vi "meas_1_lxy.vi"(0 "config":T1={"initialize"=enum."SR830", "6221"={"6221 Resource"="GPIB0::24::INSTR", "Delta status"=FALSE, "电流|RMS(A)"=0.0}, "SR830+6221"={"source"=0, "Current(A)"=0.0, "阻抗(Ohm)"=0.0, "SR830 1"=FALSE, "SR830 2"=FALSE, "SR830 3"=FALSE, "SR830 4"=FALSE, "VISA 1"="", "VISA 2"="", "VISA 3"="", "VISA 4"="", "Reserve 1"=0, "Reserve 2"=-1, "Reserve 3"=-1, "Reserve 4"=-1, "Sensitivity 1"=-1, "Sensitivity 2"=0, "Sensitivity 3"=-1, "Sensitivity 4"=-1, "量程入 1"=0, "量程入 2"=0, "量程入 3"=0, "量程入 4"=0}, "2400"={"2400"=FALSE, "VISA"="", "Output Level (0)"=1e-05, "Compliance  Level (0.1)"=10.0, "ch"=[]}, "ch"={"ch"=[], "current"=[], "change?"=[], "holding current\nwhen change ch?"=FALSE, "current offset"=[]}, "Instrument"={"limit"={"Field limit"=0.0, "Field rate limit"=0.0, "Temp limit"=0.0, "Temp low limit"=0.0, "Temp rate limit "=0.0}, "genarl"={"行数"=refnum, "编辑列表框？"=refnum, "列表框"=refnum, "camg 振荡状态"=refnum, "Aborting"=refnum, "数据文件"=refnum, "warning"=refnum, "vi路径"="", "Instrument Type"=enum."PPMS-Rotate"}, "cmag"={"TM620"="TCPIP0::192.168.1.5::4266::SOCKET", "M24C Resource"="GPIB0::24::INSTR", "4G supply"="", "Temp Status 24C"=refnum, "Temp"=refnum, "9T信号"=refnum, "4g supply status"=refnum, "in-plane"="", "out-plane"="", "in-plane signal"=FALSE, "out-plane signal"=FALSE, "in plane 信号"=refnum, "pzt volt"=refnum, "camg Rate"=refnum}, "lengtou2"={"750 visa"="", "750 rotate"="", "semaphore 340"=refnum, "semaphore 750"=refnum, "750 field status"=refnum, "Input (0:A) 340"=0, "340 Resource"="GPIB0::14::INSTR", "340 Status"=refnum, "Input (0:B) 340"=1, "Loop (0: 1)"=0, "Loop (1: 1)"=0, "TCP master instance"=refnum}, "lengtou"={"TCP master instance"=refnum, "335 Status"=refnum, "335 Resource "="GPIB0::24::INSTR", "Input (0:A) 335"=0, "Input (0:B) 335"=1, "Heater Output (1:1) 335"=1, "semaphore 335"=refnum}, "325 for test"={"quantum design"=refnum, "semaphore 325"=refnum, "325 Resource "="GPIB0::13::INSTR", "Input (0:A) 325"=0, "Heater Output (1:1) 325"=1, "325 Status"=refnum}}, "2614B"={"2614B chA"=FALSE, "2614B chB"=FALSE, "VISA"=""}, "33522b"={"33522b resource name"="", "零电压"=0.0, "最大电压"=148.0, "间隔"=4.0, "最小电压"=-48.0, "loop"=0.0, "压电陶瓷电压(Vpp)"=0.0}, "gating type"=enum."2614(daul)", "层数"=0, "行数"=0, "是否处理"=[], "current 2"=[]} {"Instrument"."325 for test"."Heater Output (1:1) 325" items=["1"=1, "2"=2]; "Instrument"."325 for test"."Input (0:A) 325" items=["A", "B"]; "Instrument"."lengtou"."Heater Output (1:1) 335" items=["1"=1, "2"=2]; "Instrument"."lengtou"."Input (0:B) 335" items=["A", "B"]; "Instrument"."lengtou"."Input (0:A) 335" items=["A", "B"]; "Instrument"."lengtou2"."Loop (1: 1)" items=["1", "2"]; "Instrument"."lengtou2"."Loop (0: 1)" items=["1", "2"]; "Instrument"."lengtou2"."Input (0:B) 340" items=["A", "B", "C", "D"]; "Instrument"."lengtou2"."Input (0:A) 340" items=["A", "B", "C", "D"]; "SR830+6221"."Sensitivity 4" items=["Auto Gain"=-1, "2 nV/fA"=0, "5 nV/fA"=1, "10 nV/fA"=2, "20 nV/fA"=3, "50 nV/fA"=4, "100 nV/fA"=5, "200 nV/fA"=6, "500 nV/fA"=7, "1 uV/pA"=8, "2 uV/pA"=9, "5 uV/pA"=10, "10 uV/pA"=11, "20 uV/pA"=12, "50 uV/pA"=13, "100 uV/pA"=14, "200 uV/pA"=15, "500 uV/pA"=16, "1 mV/nA"=17, "2 mV/nA"=18, "5 mV/nA"=19, "10 mV/nA"=20, "20 mV/nA"=21, "50 mV/nA"=22, "100 mV/nA"=23, "200 mV/nA"=24, "500 mV/mA"=25, "1 V/uA"=26]; "SR830+6221"."Sensitivity 3" items=["Auto Gain"=-1, "2 nV/fA"=0, "5 nV/fA"=1, "10 nV/fA"=2, "20 nV/fA"=3, "50 nV/fA"=4, "100 nV/fA"=5, "200 nV/fA"=6, "500 nV/fA"=7, "1 uV/pA"=8, "2 uV/pA"=9, "5 uV/pA"=10, "10 uV/pA"=11, "20 uV/pA"=12, "50 uV/pA"=13, "100 uV/pA"=14, "200 uV/pA"=15, "500 uV/pA"=16, "1 mV/nA"=17, "2 mV/nA"=18, "5 mV/nA"=19, "10 mV/nA"=20, "20 mV/nA"=21, "50 mV/nA"=22, "100 mV/nA"=23, "200 mV/nA"=24, "500 mV/mA"=25, "1 V/uA"=26]; "SR830+6221"."Sensitivity 1" items=["Auto Gain"=-1, "2 nV/fA"=0, "5 nV/fA"=1, "10 nV/fA"=2, "20 nV/fA"=3, "50 nV/fA"=4, "100 nV/fA"=5, "200 nV/fA"=6, "500 nV/fA"=7, "1 uV/pA"=8, "2 uV/pA"=9, "5 uV/pA"=10, "10 uV/pA"=11, "20 uV/pA"=12, "50 uV/pA"=13, "100 uV/pA"=14, "200 uV/pA"=15, "500 uV/pA"=16, "1 mV/nA"=17, "2 mV/nA"=18, "5 mV/nA"=19, "10 mV/nA"=20, "20 mV/nA"=21, "50 mV/nA"=22, "100 mV/nA"=23, "200 mV/nA"=24, "500 mV/mA"=25, "1 V/uA"=26]; "SR830+6221"."Sensitivity 2" items=["Auto Gain"=-1, "2 nV/fA"=0, "5 nV/fA"=1, "10 nV/fA"=2, "20 nV/fA"=3, "50 nV/fA"=4, "100 nV/fA"=5, "200 nV/fA"=6, "500 nV/fA"=7, "1 uV/pA"=8, "2 uV/pA"=9, "5 uV/pA"=10, "10 uV/pA"=11, "20 uV/pA"=12, "50 uV/pA"=13, "100 uV/pA"=14, "200 uV/pA"=15, "500 uV/pA"=16, "1 mV/nA"=17, "2 mV/nA"=18, "5 mV/nA"=19, "10 mV/nA"=20, "20 mV/nA"=21, "50 mV/nA"=22, "100 mV/nA"=23, "200 mV/nA"=24, "500 mV/mA"=25, "1 V/uA"=26]; "SR830+6221"."Reserve 4" items=["Auto Gain"=-1, "2 nV/fA"=0, "5 nV/fA"=1, "10 nV/fA"=2, "20 nV/fA"=3, "50 nV/fA"=4, "100 nV/fA"=5, "200 nV/fA"=6, "500 nV/fA"=7, "1 uV/pA"=8, "2 uV/pA"=9, "5 uV/pA"=10, "10 uV/pA"=11, "20 uV/pA"=12, "50 uV/pA"=13, "100 uV/pA"=14, "200 uV/pA"=15, "500 uV/pA"=16, "1 mV/nA"=17, "2 mV/nA"=18, "5 mV/nA"=19, "10 mV/nA"=20, "20 mV/nA"=21, "50 mV/nA"=22, "100 mV/nA"=23, "200 mV/nA"=24, "500 mV/mA"=25, "1 V/uA"=26]; "SR830+6221"."Reserve 3" items=["Auto Reserve"=-1, "High Reserve"=0, "Normal"=1, "Low Noise"=2]; "SR830+6221"."Reserve 2" items=["Auto Reserve"=-1, "High Reserve"=0, "Normal"=1, "Low Noise"=2]; "SR830+6221"."Reserve 1" items=["Auto Reserve"=-1, "High Reserve"=0, "Normal"=1, "Low Noise"=2]; "SR830+6221"."source" items=["SR830 1", "SR830 2", "SR830 3", "SR830 4"]}, 1 "压电陶瓷电压 (Vpp)":dbl=0.1, 5 "6221ch":i32, 7 "2400通道":i32, 9 "电流（A）":dbl, 11 "错误输入（无错误）":errorcluster, 12 "change？":bool) -> (4 "数组":string[](array[string]), 6 "输出簇":T1={"initialize"=enum."SR830", "6221"={"6221 Resource"="GPIB0::24::INSTR", "Delta status"=FALSE, "电流|RMS(A)"=0.0}, "SR830+6221"={"source"=0, "Current(A)"=0.0, "阻抗(Ohm)"=0.0, "SR830 1"=FALSE, "SR830 2"=FALSE, "SR830 3"=FALSE, "SR830 4"=FALSE, "VISA 1"="", "VISA 2"="", "VISA 3"="", "VISA 4"="", "Reserve 1"=0, "Reserve 2"=-1, "Reserve 3"=-1, "Reserve 4"=-1, "Sensitivity 1"=-1, "Sensitivity 2"=0, "Sensitivity 3"=-1, "Sensitivity 4"=-1, "量程入 1"=0, "量程入 2"=0, "量程入 3"=0, "量程入 4"=0}, "2400"={"2400"=FALSE, "VISA"="", "Output Level (0)"=1e-05, "Compliance  Level (0.1)"=10.0, "ch"=[]}, "ch"={"ch"=[], "current"=[], "change?"=[], "holding current\nwhen change ch?"=FALSE, "current offset"=[]}, "Instrument"={"limit"={"Field limit"=0.0, "Field rate limit"=0.0, "Temp limit"=0.0, "Temp low limit"=0.0, "Temp rate limit "=0.0}, "genarl"={"行数"=refnum, "编辑列表框？"=refnum, "列表框"=refnum, "camg 振荡状态"=refnum, "Aborting"=refnum, "数据文件"=refnum, "warning"=refnum, "vi路径"="", "Instrument Type"=enum."PPMS-Rotate"}, "cmag"={"TM620"="TCPIP0::192.168.1.5::4266::SOCKET", "M24C Resource"="GPIB0::24::INSTR", "4G supply"="", "Temp Status 24C"=refnum, "Temp"=refnum, "9T信号"=refnum, "4g supply status"=refnum, "in-plane"="", "out-plane"="", "in-plane signal"=FALSE, "out-plane signal"=FALSE, "in plane 信号"=refnum, "pzt volt"=refnum, "camg Rate"=refnum}, "lengtou2"={"750 visa"="", "750 rotate"="", "semaphore 340"=refnum, "semaphore 750"=refnum, "750 field status"=refnum, "Input (0:A) 340"=0, "340 Resource"="GPIB0::14::INSTR", "340 Status"=refnum, "Input (0:B) 340"=1, "Loop (0: 1)"=0, "Loop (1: 1)"=0, "TCP master instance"=refnum}, "lengtou"={"TCP master instance"=refnum, "335 Status"=refnum, "335 Resource "="GPIB0::24::INSTR", "Input (0:A) 335"=0, "Input (0:B) 335"=1, "Heater Output (1:1) 335"=1, "semaphore 335"=refnum}, "325 for test"={"quantum design"=refnum, "semaphore 325"=refnum, "325 Resource "="GPIB0::13::INSTR", "Input (0:A) 325"=0, "Heater Output (1:1) 325"=1, "325 Status"=refnum}}, "2614B"={"2614B chA"=FALSE, "2614B chB"=FALSE, "VISA"=""}, "33522b"={"33522b resource name"="", "零电压"=0.0, "最大电压"=148.0, "间隔"=4.0, "最小电压"=-48.0, "loop"=0.0, "压电陶瓷电压(Vpp)"=0.0}, "gating type"=enum."2614(daul)", "层数"=0, "行数"=0, "是否处理"=[], "current 2"=[]} {"Instrument"."325 for test"."Heater Output (1:1) 325" items=["1"=1, "2"=2]; "Instrument"."325 for test"."Input (0:A) 325" items=["A", "B"]; "Instrument"."lengtou"."Heater Output (1:1) 335" items=["1"=1, "2"=2]; "Instrument"."lengtou"."Input (0:B) 335" items=["A", "B"]; "Instrument"."lengtou"."Input (0:A) 335" items=["A", "B"]; "Instrument"."lengtou2"."Loop (1: 1)" items=["1", "2"]; "Instrument"."lengtou2"."Loop (0: 1)" items=["1", "2"]; "Instrument"."lengtou2"."Input (0:B) 340" items=["A", "B", "C", "D"]; "Instrument"."lengtou2"."Input (0:A) 340" items=["A", "B", "C", "D"]; "SR830+6221"."Sensitivity 4" items=["Auto Gain"=-1, "2 nV/fA"=0, "5 nV/fA"=1, "10 nV/fA"=2, "20 nV/fA"=3, "50 nV/fA"=4, "100 nV/fA"=5, "200 nV/fA"=6, "500 nV/fA"=7, "1 uV/pA"=8, "2 uV/pA"=9, "5 uV/pA"=10, "10 uV/pA"=11, "20 uV/pA"=12, "50 uV/pA"=13, "100 uV/pA"=14, "200 uV/pA"=15, "500 uV/pA"=16, "1 mV/nA"=17, "2 mV/nA"=18, "5 mV/nA"=19, "10 mV/nA"=20, "20 mV/nA"=21, "50 mV/nA"=22, "100 mV/nA"=23, "200 mV/nA"=24, "500 mV/mA"=25, "1 V/uA"=26]; "SR830+6221"."Sensitivity 3" items=["Auto Gain"=-1, "2 nV/fA"=0, "5 nV/fA"=1, "10 nV/fA"=2, "20 nV/fA"=3, "50 nV/fA"=4, "100 nV/fA"=5, "200 nV/fA"=6, "500 nV/fA"=7, "1 uV/pA"=8, "2 uV/pA"=9, "5 uV/pA"=10, "10 uV/pA"=11, "20 uV/pA"=12, "50 uV/pA"=13, "100 uV/pA"=14, "200 uV/pA"=15, "500 uV/pA"=16, "1 mV/nA"=17, "2 mV/nA"=18, "5 mV/nA"=19, "10 mV/nA"=20, "20 mV/nA"=21, "50 mV/nA"=22, "100 mV/nA"=23, "200 mV/nA"=24, "500 mV/mA"=25, "1 V/uA"=26]; "SR830+6221"."Sensitivity 1" items=["Auto Gain"=-1, "2 nV/fA"=0, "5 nV/fA"=1, "10 nV/fA"=2, "20 nV/fA"=3, "50 nV/fA"=4, "100 nV/fA"=5, "200 nV/fA"=6, "500 nV/fA"=7, "1 uV/pA"=8, "2 uV/pA"=9, "5 uV/pA"=10, "10 uV/pA"=11, "20 uV/pA"=12, "50 uV/pA"=13, "100 uV/pA"=14, "200 uV/pA"=15, "500 uV/pA"=16, "1 mV/nA"=17, "2 mV/nA"=18, "5 mV/nA"=19, "10 mV/nA"=20, "20 mV/nA"=21, "50 mV/nA"=22, "100 mV/nA"=23, "200 mV/nA"=24, "500 mV/mA"=25, "1 V/uA"=26]; "SR830+6221"."Sensitivity 2" items=["Auto Gain"=-1, "2 nV/fA"=0, "5 nV/fA"=1, "10 nV/fA"=2, "20 nV/fA"=3, "50 nV/fA"=4, "100 nV/fA"=5, "200 nV/fA"=6, "500 nV/fA"=7, "1 uV/pA"=8, "2 uV/pA"=9, "5 uV/pA"=10, "10 uV/pA"=11, "20 uV/pA"=12, "50 uV/pA"=13, "100 uV/pA"=14, "200 uV/pA"=15, "500 uV/pA"=16, "1 mV/nA"=17, "2 mV/nA"=18, "5 mV/nA"=19, "10 mV/nA"=20, "20 mV/nA"=21, "50 mV/nA"=22, "100 mV/nA"=23, "200 mV/nA"=24, "500 mV/mA"=25, "1 V/uA"=26]; "SR830+6221"."Reserve 4" items=["Auto Gain"=-1, "2 nV/fA"=0, "5 nV/fA"=1, "10 nV/fA"=2, "20 nV/fA"=3, "50 nV/fA"=4, "100 nV/fA"=5, "200 nV/fA"=6, "500 nV/fA"=7, "1 uV/pA"=8, "2 uV/pA"=9, "5 uV/pA"=10, "10 uV/pA"=11, "20 uV/pA"=12, "50 uV/pA"=13, "100 uV/pA"=14, "200 uV/pA"=15, "500 uV/pA"=16, "1 mV/nA"=17, "2 mV/nA"=18, "5 mV/nA"=19, "10 mV/nA"=20, "20 mV/nA"=21, "50 mV/nA"=22, "100 mV/nA"=23, "200 mV/nA"=24, "500 mV/mA"=25, "1 V/uA"=26]; "SR830+6221"."Reserve 3" items=["Auto Reserve"=-1, "High Reserve"=0, "Normal"=1, "Low Noise"=2]; "SR830+6221"."Reserve 2" items=["Auto Reserve"=-1, "High Reserve"=0, "Normal"=1, "Low Noise"=2]; "SR830+6221"."Reserve 1" items=["Auto Reserve"=-1, "High Reserve"=0, "Normal"=1, "Low Noise"=2]; "SR830+6221"."source" items=["SR830 1", "SR830 2", "SR830 3", "SR830 4"]}, 15 "错误输出":errorcluster)   [LabVIEW 2019, in "nematic.lvlib"]
uses:
  nematic.lvlib
  ctl/config.ctl
  <vilib>/NI/Modbus Library/API/Master/Modbus Master.lvclass
  ctl/initialize.ctl
  ctl/Instrument.ctl
  ctl/limit.ctl
  ctl/warning.ctl
  ctl/Instrument Type.ctl
  ctl/335 state.ctl
  ctl/9T mag field stauts.ctl
  C:/Users/fuyang/Desktop/postdoctor/labview/labview-measure/lib/QDInstrument.dll
  lib/QDInstrument.dll
  ctl/Gating type.ctl
  lib/Keithley 622x/Configure/Format/Typedefs/KE622x -- Optional Meas Elements.ctl
  <vilib>/Analysis/baseanly.llb/Mean (DBL).vi
  SubVI.lvlib
  Get value.lvlib
  lib/Keithley 622x/Keithley 622x.lvlib
  <vilib>/Analysis/NI_AALBase.lvlib
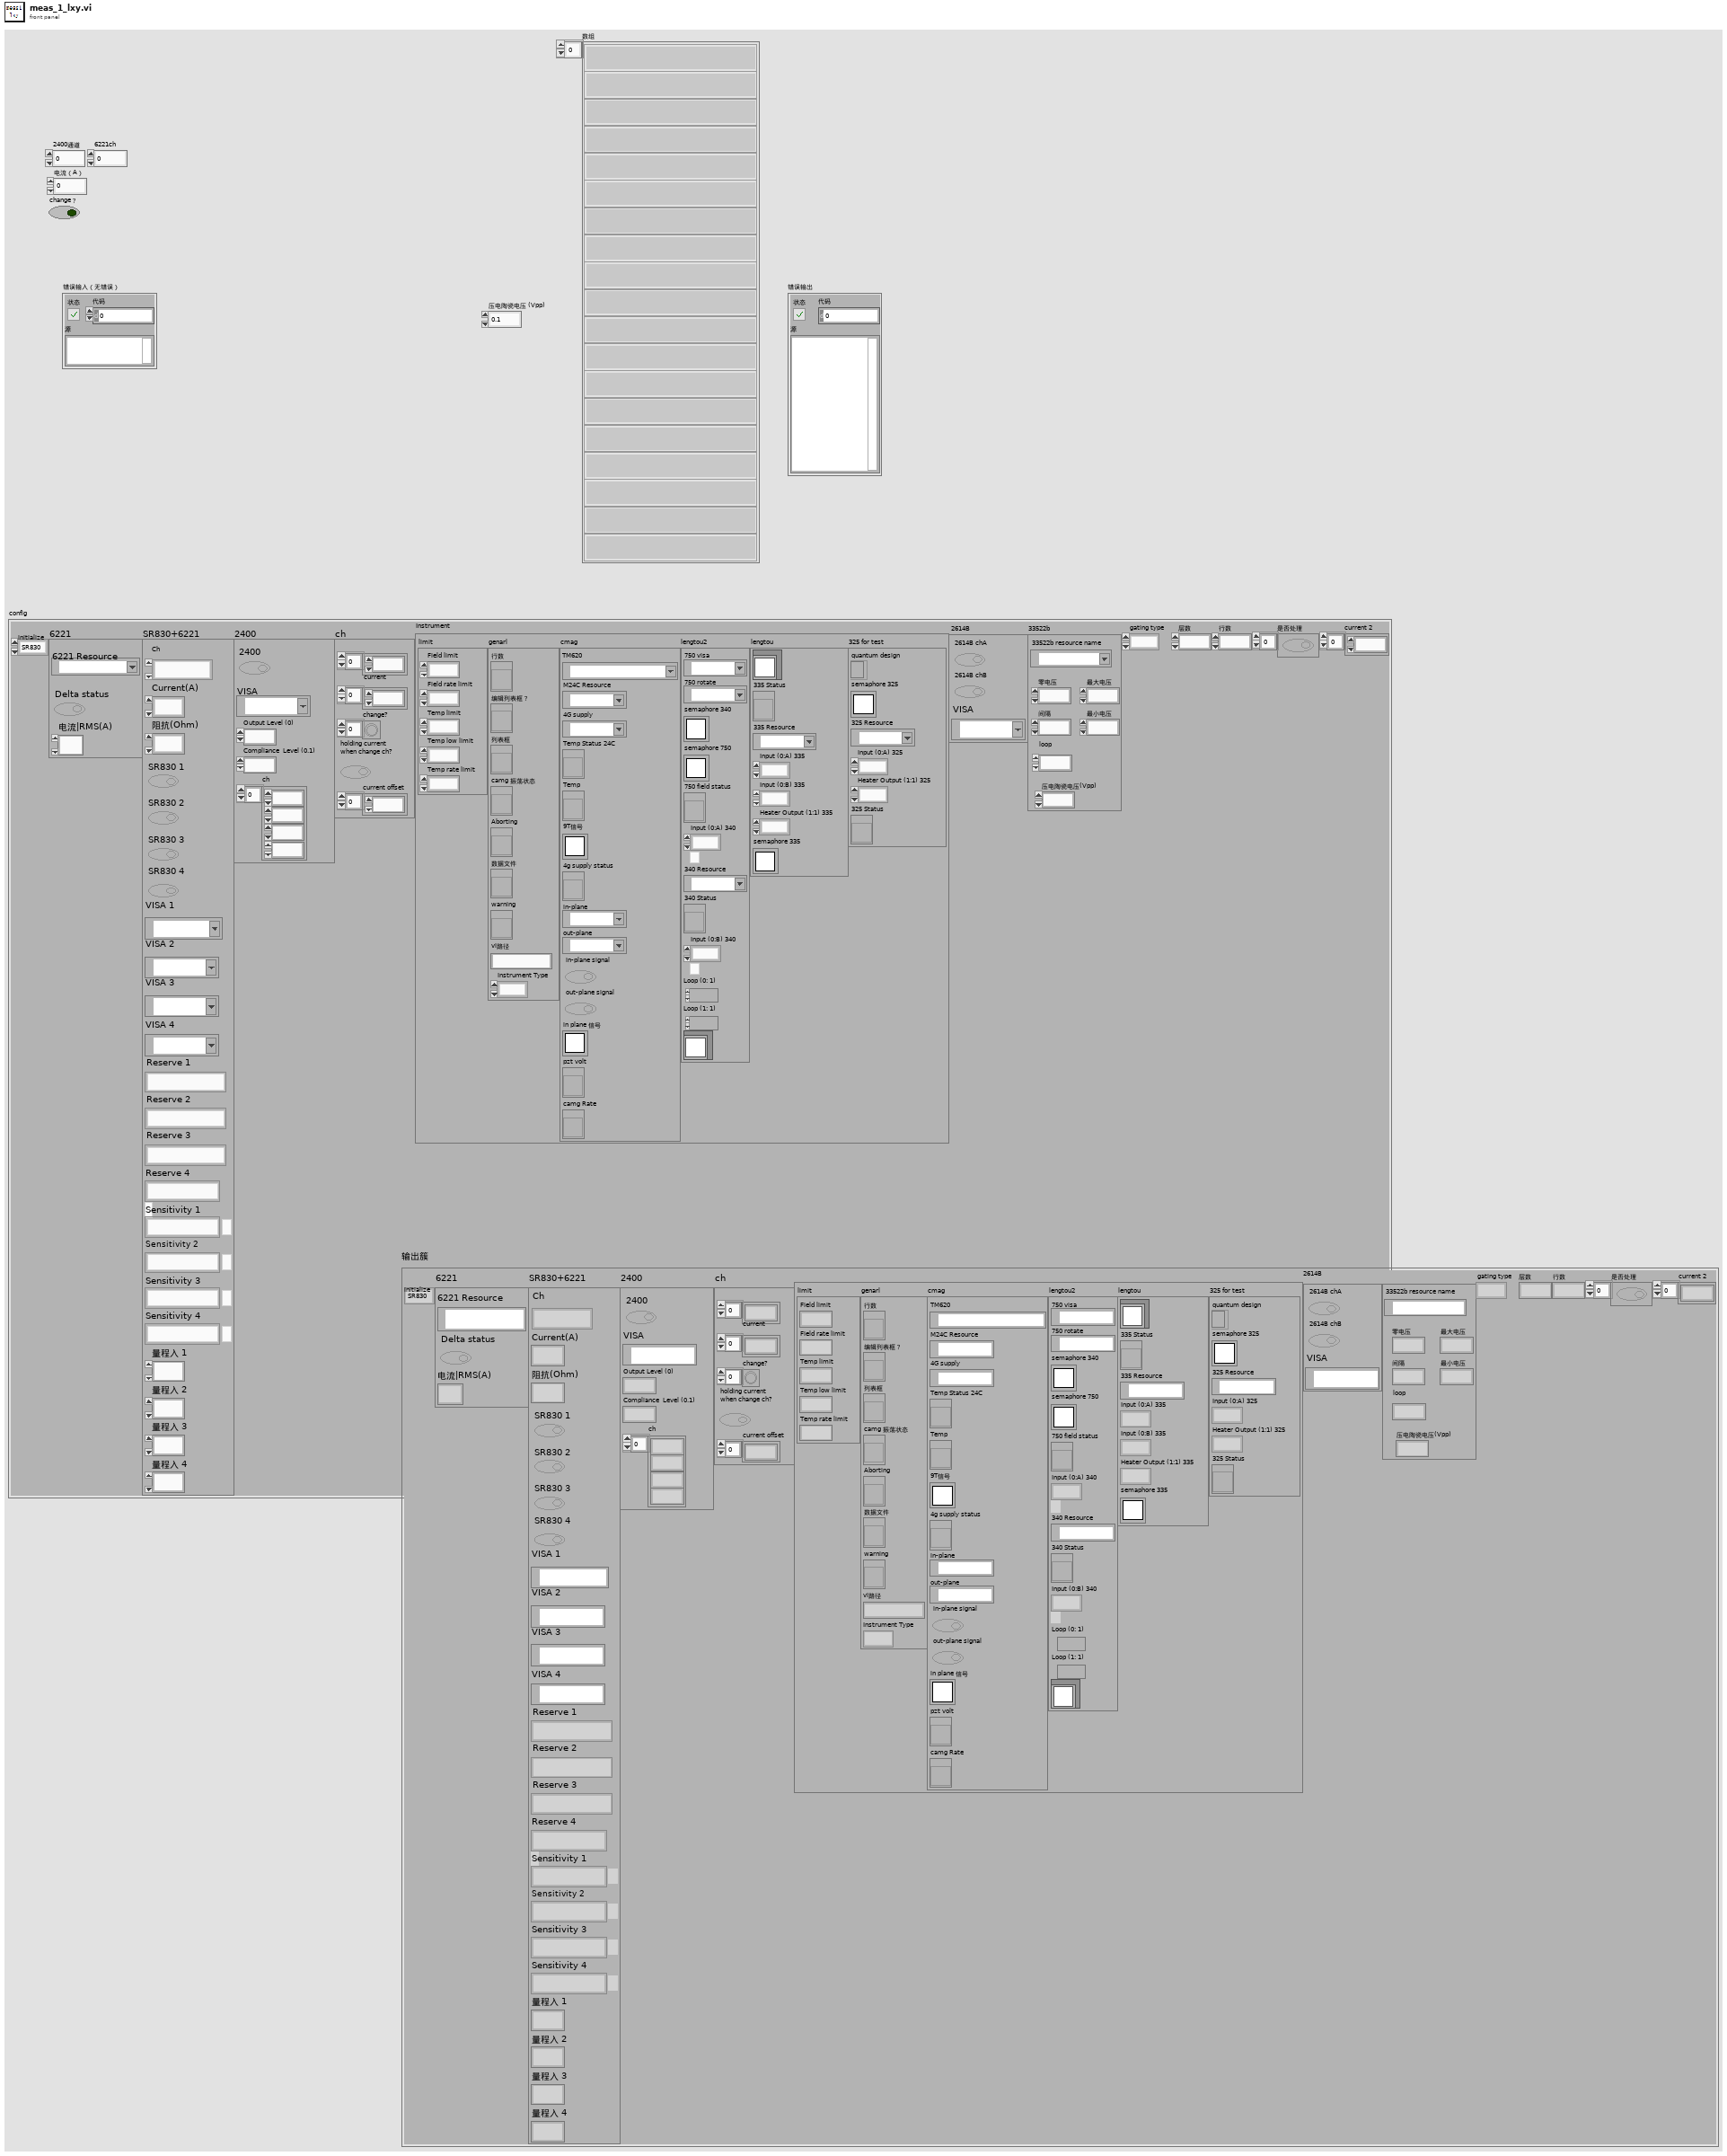
[diagram p1: front panel]
types:
  T1 = typedef "config.ctl" = cluster{"initialize":T2, "6221":cluster{"6221 Resource":refnum<visa-resource-name>, "Delta status":bool, "电流|RMS(A)":dbl}, "SR830+6221":cluster{"source":u16, "Current(A)":dbl, "阻抗(Ohm)":dbl, "SR830 1":bool, "SR830 2":bool, "SR830 3":bool, "SR830 4":bool, "VISA 1":refnum<visa-resource-name>, "VISA 2":refnum<visa-resource-name>, "VISA 3":refnum<visa-resource-name>, "VISA 4":refnum<visa-resource-name>, "Reserve 1":i16, "Reserve 2":i16, "Reserve 3":i16, "Reserve 4":i16, "Sensitivity 1":i16, "Sensitivity 2":i16, "Sensitivity 3":i16, "Sensitivity 4":i16, "量程入 1":i32, "量程入 2":i32, "量程入 3":i32, "量程入 4":i32}, "2400":cluster{"2400":bool, "VISA":refnum<visa-resource-name>, "Output Level (0)":dbl, "Compliance  Level (0.1)":dbl, "ch":i32[]}, "ch":cluster{"ch":i32[], "current":dbl[], "change?":bool[], "holding current\nwhen change ch?":bool, "current offset":dbl[]}, "Instrument":T3, "2614B":cluster{"2614B chA":bool, "2614B chB":bool, "VISA":refnum<visa-resource-name>}, "33522b":cluster{"33522b resource name":refnum<visa-resource-name>, "零电压":dbl, "最大电压":dbl, "间隔":dbl, "最小电压":dbl, "loop":dbl, "压电陶瓷电压(Vpp)":dbl}, "gating type":T7, "层数":i32, "行数":i32, "是否处理":bool[], "current 2":dbl[]}
  T2 = typedef "initialize.ctl" = enum16{"SR830", "keithley6221-SR830", "Delta", "Delta-tunnelling", "keithley6221-2182-DC", "PZT", "4200"}
  T3 = typedef "Instrument.ctl" = cluster{"limit":T4, "genarl":cluster{"行数":refnum<vi>, "编辑列表框？":refnum<vi>, "列表框":refnum<vi>, "camg 振荡状态":refnum<vi>, "Aborting":refnum<vi>, "数据文件":refnum<vi>, "warning":refnum<vi>, "vi路径":string, "Instrument Type":T5}, "cmag":cluster{"TM620":refnum<visa-resource-name>, "M24C Resource":refnum<visa-resource-name>, "4G supply":refnum<visa-resource-name>, "Temp Status 24C":refnum<vi>, "Temp":refnum<vi>, "9T信号":T6, "4g supply status":refnum<vi>, "in-plane":refnum<visa-resource-name>, "out-plane":refnum<visa-resource-name>, "in-plane signal":bool, "out-plane signal":bool, "in plane 信号":T6, "pzt volt":refnum<vi>, "camg Rate":refnum<vi>}, "lengtou2":cluster{"750 visa":refnum<visa-resource-name>, "750 rotate":refnum<visa-resource-name>, "semaphore 340":T6, "semaphore 750":T6, "750 field status":refnum<vi>, "Input (0:A) 340":u16, "340 Resource":refnum<visa-resource-name>, "340 Status":refnum<vi>, "Input (0:B) 340":u16, "Loop (0: 1)":u16, "Loop (1: 1)":u16, "TCP master instance":refnum<class "Modbus Master.lvclass">}, "lengtou":cluster{"TCP master instance":refnum<class "Modbus Master.lvclass">, "335 Status":refnum<vi>, "335 Resource ":refnum<visa-resource-name>, "Input (0:A) 335":u16, "Input (0:B) 335":u16, "Heater Output (1:1) 335":u16, "semaphore 335":T6}, "325 for test":cluster{"quantum design":refnum<k24>, "semaphore 325":T6, "325 Resource ":refnum<visa-resource-name>, "Input (0:A) 325":u16, "Heater Output (1:1) 325":u16, "325 Status":refnum<vi>}}
  T4 = typedef "limit.ctl" = cluster{"Field limit":dbl, "Field rate limit":dbl, "Temp limit":dbl, "Temp low limit":dbl, "Temp rate limit ":dbl}
  T5 = typedef "Instrument Type.ctl" = enum16{"PPMS", "VersaLab", "DynaCool", "SVSM", "PPMS-Rotate", "Lakeshore335", "lengtou2", "9T mag old", "9T cmag", "9T cmag DAC", "9T cmag rotate", "test"}
  T6 = typedef "Semaphore RefNum" = refnum<k1>
  T7 = typedef "Gating type.ctl" = enum32{"null", "2614(daul)", "2400", "6517B"}
  T8 = typedef "Keithley 622x.lvlib/KE622x -- Optional Meas Elements.ctl" = cluster{"Timstamp?":bool, "Reading Num?":bool, "Source Value?":bool, "Compliance?":bool, "Average Voltage?":bool}
  T9 = typedef "Keithley 622x.lvlib/KE622x -- Meas Event Reg State.ctl" = cluster{"B0, ROF:  KE2182A Delta Reading Overflow Event?":bool, "B1, Int:  Interlock OK Event?":bool, "B2, Temp:  Over Temperature Event?":bool, "B3, Comp:  Compliance Event?":bool, "B5, RAV:  Delta Reading Available Event?":bool, "B6, TN:  User Defined Reading Number Stored In Buffer Event?":bool, "B7, BAV:  At Least 2 Readings Stored In Buffer Event?":bool, "B12, BQF:  Buffer Quarter Full Event?":bool, "B8, BHF:  Buffer Half Full Event?":bool, "B13, B3QF:  Buffer 3/4 Full Event?":bool, "B9, BFL:  Buffer Full Event?":bool}
  T10 = typedef "Keithley 622x.lvlib/KE622x -- Trace Buf.ctl" = cluster{"Additional Valid Arrays":T8, "Reading Num":u32[], "Timestamp (secs)":sgl[], "Source Val (A)":sgl[], "Reading":sgl[], "Average Voltage (V)":sgl[], "Compliance?":bool[]}
  T11 = typedef "warning.ctl" = cluster{"Compliance":bool}
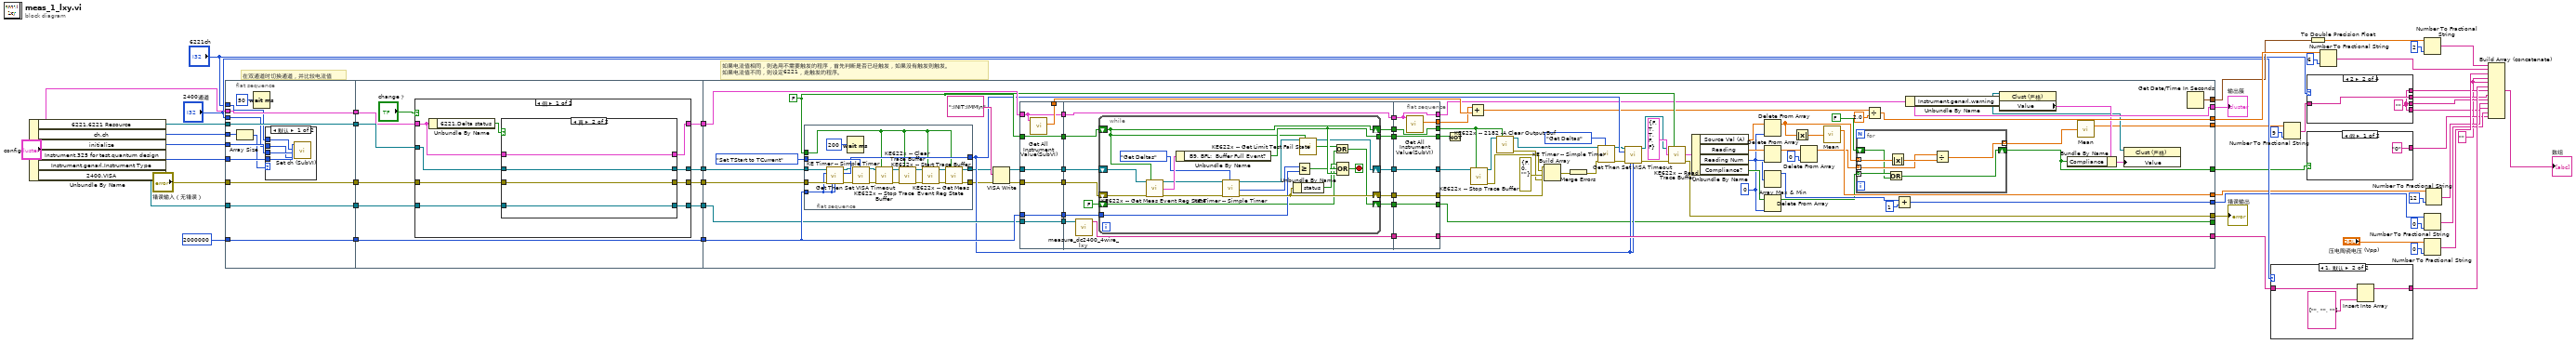
[diagram p0: block diagram]
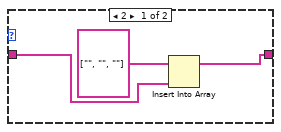
[diagram p2: hidden frame]
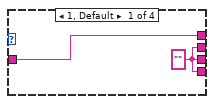
[diagram p3: hidden frame]
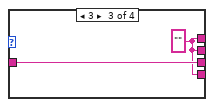
[diagram p4: hidden frame]
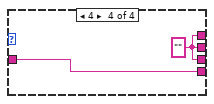
[diagram p5: hidden frame]
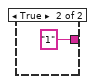
[diagram p6: hidden frame]
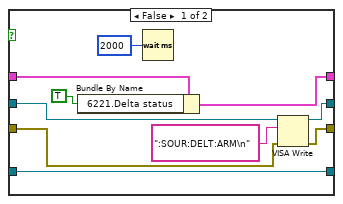
[diagram p8: hidden frame]
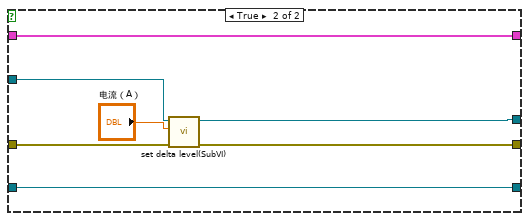
[diagram p9: hidden frame]
diagram:
  w2 = "" ("元素")
  # "如果电流值相同，则选用不需要触发的程序，首先判断是否已经触发，如果没有触发则触发。\n如果电流值不同，则设定6221，走触发的程序。"
  # "在双通道时切换通道，并比较电流值"
  n1 = Unbundle By Name("config") -> ("6221.6221 Resource"=w38:refnum<visa-resource-name>, "ch.ch"=w26:i32[], "initialize"=w36:T2, "Instrument.genarl.Instrument Type"=w35:T5, "2400.VISA"=w39:refnum<visa-resource-name>)  [unwired: 1 out]
  n2 = flat-sequence {
    tunnel: w39 -> [w60]
    tunnel: "错误输入（无错误）" -> [w61]
    tunnel: w38 -> [w62]
    tunnel: u32 2000000 ("Timeout (20000 ms)") -> [w63]
    tunnel: [w63] -> w44
    tunnel: [w62] -> w43
    tunnel: [w61] -> w42
    tunnel: [w60] -> w41
    tunnel: "config" -> [w59]
    tunnel: [w59] -> w40
    tunnel: w26 -> [w57]
    tunnel: w36 -> [w56]
    tunnel: w35 -> [w55]
    tunnel: "2400通道" -> [w53]
    tunnel: "6221ch" -> [w52]
    tunnel: w44 -> [w77]
    tunnel: [w77] -> w31
    tunnel: w43 -> [w76]
    tunnel: [w75] -> w30
    tunnel: w42 -> [w72]
    tunnel: [w70] -> w29
    tunnel: w41 -> [w74]
    tunnel: [w73] -> w28
    tunnel: w40 -> [w71]
    tunnel: [w69] -> w25
    tunnel: w31 -> [w183]
    tunnel: w30 -> [w181]
    tunnel: w29 -> [w182]
    tunnel: w28 -> [w180]
    tunnel: [w179] -> w16
    tunnel: [w178] -> w27
    tunnel: w25 -> [w175]
    tunnel: [w177] -> w24
    tunnel: [w176] -> w23
    tunnel: [w113] -> w22
    tunnel: [w174] -> w19
    tunnel: [w173] -> w14
    tunnel: [w117] -> _
    tunnel: [w109] -> w13
    tunnel: [w108] -> w6
    frame #0 {
      n3 = Array Size(array=w57) -> (size(s)=w54:i32)
      n4 = Wait (ms)(milliseconds to wait=u32 50) -> ()  [unwired: 1 out]
      n5 = case shown="默认" w54 {
        tunnel: w55 -> [w67 _]
        tunnel: w56 -> [w66 _]
        tunnel: w53 -> [w65 _]
        tunnel: w52 -> [w64 _]
        frame Default {
          n6 = call "Set ch (SubVI).vi"("2400通道"=w65, "initialize"=w66, "数值"=w64, "Instrument Type"=w67) -> ()  [unwired: 8 in]
        }
        frame 0, 1 {
        }
      }
    }
    frame #1 {
      n7 = case shown="假" "change？" {
        tunnel: w72 -> [w85 w107]
        tunnel: w76 -> [w86 w106]
        tunnel: [w84 w105] -> w75
        tunnel: [w83 w104] -> w70
        tunnel: w74 -> [w78 w103]
        tunnel: [w79 w103] -> w73
        tunnel: w71 -> [w81 w102]
        tunnel: [w80 w102] -> w69
        frame False {
          n8 = Unbundle By Name(w81) -> ("6221.Delta status"=w82:bool)
          n9 = case shown="真" w82 {
            tunnel: w86 -> [w92 w99]
            tunnel: [w93 w99] -> w84
            tunnel: w85 -> [w95 w100]
            tunnel: [w94 w100] -> w83
            tunnel: w81 -> [w89 w98]
            tunnel: [w88 w98] -> w80
            tunnel: w78 -> [w87 w97]
            tunnel: [w87 w97] -> w79
            frame False {
              n10 = Bundle By Name(cluster=w89, "6221.Delta status"=TRUE) -> (w88:T1)
              n11 = Wait (ms)(milliseconds to wait=u32 2000) -> ()  [unwired: 1 out]
              n12 = VISA Write(VISA resource name=w92, write buffer=":SOUR:DELT:ARM\n" ("format string"), error in (no error)=w95) -> (VISA resource name out=w93:refnum<visa-resource-name>, error out=w94:errorcluster)  [unwired: 1 out]
            }
            frame True {
            }
          }
        }
        frame True {
          n13 = call "set delta level(SubVI).vi"("错误输入（无错误）"=w107, "电流（A）"="电流（A）", "VISA引用句柄输入"=w106) -> ("错误输出"=w104:errorcluster, "VISA引用句柄输出"=w105:refnum<visa-resource-name>)  [unwired: 7 in]
        }
      }
    }
    frame #2 {
      w154 = FALSE ("Check For SCPI Errors? (T) 2")
      w126 = 0 ("索引")
      n14 = flat-sequence {
        tunnel: enum16{"Set TStart to TCurrent", "Get Deltas"}."Set TStart to TCurrent" ("Action") -> [w252]
        tunnel: [w239] -> w137
        tunnel: [w238] -> w138
        tunnel: [w247] -> w145
        tunnel: w181 -> [w244]
        tunnel: w154 -> [w243]
        tunnel: w182 -> [w242]
        tunnel: w183 -> [w241]
        frame #0 {
          n15 = call "Get Then Set VISA Timeout.vi"("VISA Resource Name In"=w244, "New Timeout (msecs)"=w241, "error in (no error)"=w242, "Max Timeout (300 secs)"=w241, "Min Timeout (3 secs)"=w241) -> ("VISA Resource Name Out (dupl)"=w246:refnum<visa-resource-name>, "Old Timeout (msecs)"=w247:u32, "error out"=w245:errorcluster)  [unwired: 7 in, 1 out]
          n16 = Wait (ms)(milliseconds to wait=u32 200) -> ()  [unwired: 1 out]
          n17 = call "KE Timer -- Simple Timer.vi"("Resource In"=w246, "error in (no error)"=w245, "Action"=w252) -> ("Resource Out (dupl)"=w251:refnum<visa-resource-name>, "error out (dupl)"=w250:errorcluster)  [unwired: 7 in, 8 out]
          n18 = call "KE622x -- Stop Trace Buffer.vi"("Resource In"=w251, "Check For SCPI Errors? (T)"=w243, "error in (no error)"=w250) -> ("Resource Out (dupl)"=w256:refnum<visa-resource-name>, "error out"=w255:errorcluster)  [unwired: 11 in]
          n19 = call "KE622x -- Clear Trace Buffer.vi"("Resource In"=w256, "Check For SCPI Errors? (T)"=w243, "error in (no error)"=w255) -> ("Resource Out (dupl)"=w249:refnum<visa-resource-name>, "error out"=w248:errorcluster)  [unwired: 11 in]
          n20 = call "KE622x -- Start Trace Buffer.vi"("Resource In"=w249, "Check For SCPI Errors? (T)"=w243, "error in (no error)"=w248) -> ("Resource Out (dupl)"=w253:refnum<visa-resource-name>, "error out"=w254:errorcluster)  [unwired: 11 in]
          n21 = call "KE622x -- Get Meas Event Reg State.vi"("VISA Resource In"=w253, "Error Query (T)?"=w243, "error in (no error)"=w254) -> ("VISA Resource Out (dupl)"=w239:refnum<visa-resource-name>, "error out"=w238:errorcluster)  [unwired: 10 in, 1 out]
        }
      }
      n22 = VISA Write(VISA resource name=w137, write buffer=":INIT:IMM\n", error in (no error)=w138) -> (VISA resource name out=w153:refnum<visa-resource-name>, error out=w152:errorcluster)  [unwired: 1 out]
      n23 = flat-sequence {
        tunnel: w152 -> [w193]
        tunnel: w153 -> [w194]
        tunnel: w154 -> [w195]
        tunnel: w183 -> [w196]
        tunnel: w180 -> [w197]
        tunnel: [w197] -> w172
        tunnel: [w196] -> w171
        tunnel: [w195] -> w170
        tunnel: [w194] -> w169
        tunnel: [w193] -> w168
        tunnel: [w192] -> w132
        tunnel: w175 -> [w191]
        tunnel: [w191] -> w167
        tunnel: w172 -> [w200]
        tunnel: w171 -> [w202]
        tunnel: w170 -> [w208]
        tunnel: w169 -> [w209]
        tunnel: w168 -> [w210]
        tunnel: [w199] -> w166
        tunnel: [w203] -> w165
        tunnel: [w204] -> w164
        tunnel: [w205] -> w163
        tunnel: [w206] -> w162
        tunnel: [w207] -> w161
        tunnel: [w198] -> w160
        tunnel: w167 -> [w198]
        tunnel: [w232] -> w155
        tunnel: [w233] -> w156
        tunnel: [w234] -> w157
        tunnel: [w235] -> w158
        tunnel: [w236] -> w117
        tunnel: [w237] -> w179
        tunnel: w166 -> [w237]
        tunnel: w165 -> [w236]
        tunnel: w164 -> [w235]
        tunnel: w163 -> [w234]
        tunnel: w162 -> [w233]
        tunnel: w161 -> [w232]
        tunnel: [w231] -> w131
        tunnel: w160 -> [w230]
        tunnel: [w230] -> w113
        frame #0 {
          n24 = call "Get All Instrument Value(SubVI).vi"("输出簇."=w191) -> ("数组"=w192:dbl[])  [unwired: 10 in]
        }
        frame #1 {
          n25 = call "measure_dc2400_4wire_lxy.vi"("2400 resource name"=w200) -> ("输出数组"=w199:string[])  [unwired: 8 in, 2 out]
          n26 = while {
            shift-right: [w220] -> w207
            shift-left: w210 -> [w229]
            shift-right: [w216] -> w206
            shift-left: w209 -> [w228]
            tunnel: [w222] -> w205
            shift-right: [w212] -> w204
            shift-left: w208 -> [w212]
            tunnel: w202 -> [w218]
            shift-right: [w214] -> w203
            shift-left: FALSE -> [w213]
            stop <- w211 stop-if-true
            n27 = call "KE622x -- Get Meas Event Reg State.vi"("VISA Resource In"=w228, "Error Query (T)?"=w212, "error in (no error)"=w229) -> ("VISA Resource Out (dupl)"=w225:refnum<visa-resource-name>, "KE622x Meas Event Reg"=w227:T9, "error out"=w226:errorcluster)  [unwired: 10 in]
            n28 = Unbundle By Name(w227) -> ("B9, BFL:  Buffer Full Event?"=w222:bool)
            n29 = call "KE Timer -- Simple Timer.vi"("Resource In"=w225, "error in (no error)"=w226, "Action"=enum16{"Set TStart to TCurrent", "Get Deltas"}."Get Deltas") -> ("Resource Out (dupl)"=w217:refnum<visa-resource-name>, "TCurrent - TStart (ms)"=w223:u32, "error out (dupl)"=w220:errorcluster)  [unwired: 7 in, 7 out]
            n30 = Unbundle By Name(w220) -> ("status"=w219:bool)
            n31 = Greater Or Equal?(x=w223, y=w218) -> (x >= y?=w221:bool)
            n32 = call "KE622x -- Get Limit Test Fail State.vi"("Resource In"=w217, "Check For SCPI Errors? (T)"=w212) -> ("Resource Out (dupl)"=w216:refnum<visa-resource-name>, "Limit Test Failed (Compliance)?"=w215:bool)  [unwired: 11 in, 1 out]
            n33 = Or(x=w215, y=w213) -> (x .or. y?=w214:bool)
            n34 = Compound Arithmetic op=OR(w219, w221, w222) -> (w211:bool)
          }
        }
        frame #2 {
          n35 = call "Get All Instrument Value(SubVI).vi"("输出簇."=w230) -> ("数组"=w231:dbl[])  [unwired: 10 in]
        }
      }
      n36 = Not(x=w157) -> ()  [unwired: 1 out]
      n37 = Add(x=w131, y=w132) -> (x+y=w130:dbl[])
      n38 = call "KE622x -- Stop Trace Buffer.vi"("Resource In"=w156, "Check For SCPI Errors? (T)"=w158) -> ("Resource Out (dupl)"=w148:refnum<visa-resource-name>, "error out"=w140:errorcluster)  [unwired: 12 in]
      n39 = call "KE622x -- 2182 -A Clear Output Buf.vi"("622x Resource In"=w148, "Check For SCPI Errors? (T)"=w158) -> ("622x Resource Out (dupl)"=w135:refnum<visa-resource-name>, "error out"=w141:errorcluster)  [unwired: 11 in, 1 out]
      n40 = Build Array(w155, w140, errorcluster {"status"=FALSE, "code"=0, "source"=""} ("error out"), w141) -> (w139:errorcluster[])
      n41 = Merge Errors(w139) -> (w142:errorcluster)
      n42 = call "KE Timer -- Simple Timer.vi"("Resource In"=w135, "error in (no error)"=w142, "Action"=enum16{"Set TStart to TCurrent", "Get Deltas"}."Get Deltas") -> ("Resource Out (dupl)"=w144:refnum<visa-resource-name>, "error out (dupl)"=w143:errorcluster)  [unwired: 7 in, 8 out]
      n43 = call "Get Then Set VISA Timeout.vi"("VISA Resource Name In"=w144, "New Timeout (msecs)"=w145, "error in (no error)"=w143, "Max Timeout (300 secs)"=w145, "Min Timeout (3 secs)"=w145) -> ("VISA Resource Name Out (dupl)"=w146:refnum<visa-resource-name>, "error out"=w147:errorcluster)  [unwired: 7 in, 2 out]
      n44 = call "KE622x -- Read Trace Buffer.vi"("Resource In"=w146, "Check For SCPI Errors? (T)"=w154, "Meas Elements To Return"=T8 {"Timstamp?"=FALSE, "Reading Num?"=TRUE, "Source Value?"=TRUE, "Compliance?"=FALSE, "Average Voltage?"=FALSE}, "error in (no error)"=w147) -> ("Trace Buf"=w133:T10, "error out"=w176:errorcluster)  [unwired: 9 in, 1 out]
      n45 = Unbundle By Name(w133) -> ("Source Val (A)"=w128:sgl[], "Reading"=w151:sgl[], "Reading Num"=w125:u32[], "Compliance?"=w127:bool[])
      n46 = Delete From Array(array=w128, index=w126) -> (array with subset deleted=w118:sgl[])  [unwired: 1 in, 1 out]
      n47 = Delete From Array(array=w151, index=w126) -> (array with subset deleted=w121:sgl[])  [unwired: 1 in, 1 out]
      n48 = Array Max & Min(array=w125) -> (max value=w124:u32)  [unwired: 3 out]
      n49 = Delete From Array(array=w127, index=w126) -> (array with subset deleted=w115:bool[])  [unwired: 1 in, 1 out]
      n50 = Absolute Value(x=w118) -> (abs(x)=w122:sgl[])
      n51 = Delete From Array(array=w121, index=0) -> (array with subset deleted=w119:sgl[])  [unwired: 1 in, 1 out]
      n52 = call-poly <vilib>:"Mean.vi"("X"=w122) -> ("mean"=w173:dbl)  [unwired: 1 out]
      n53 = for {
        tunnel: w119 -> [w188] mode=indexing
        tunnel: w118 -> [w190] mode=indexing
        tunnel: [w187] -> w116 mode=indexing
        tunnel: w115 -> [w185] mode=indexing
        shift-right: [w186] -> w108
        shift-left: FALSE -> [w184]
        n54 = Or(x=w185, y=w184) -> (x .or. y?=w186:bool)
        n55 = Absolute Value(x=w190) -> (abs(x)=w189:sgl)
        n56 = Divide(x=w188, y=w189) -> (x/y=w187:sgl)
      }
      n57 = Divide(x=w130, y=2.0) -> (x/y=w178:dbl[])
      n58 = Add(x=w124, y=u32 1) -> (x+y=w174:u32)
      n59 = Unbundle By Name(w113) -> ("Instrument.genarl.warning"=w110:refnum<vi>)
      n60 = property class="Clust (严格)"(reference=w110) -> ("Value"=w112:T11)  [unwired: 1 in, 2 out]
      n61 = Bundle By Name(cluster=w112, "Compliance"=w108) -> (w111:T11)
      n62 = call-poly <vilib>:"Mean.vi"("X"=w116) -> ("mean"=w109:dbl)  [unwired: 1 out]
      n63 = property class="Clust (严格)"(reference=w110, "Value"=w111) -> ()  [unwired: 1 in, 2 out]
      n64 = Get Date/Time In Seconds() -> (seconds since 1Jan1904=w177:timestamp)
    }
  }
  n65 = case shown="1, 默认" "2400通道" {
    tunnel: w16 -> [w258 w262]
    tunnel: [w257 w261] -> w15
    frame 2 {
      n66 = Insert Into Array(array=string[] ["", "", ""] ("输出数组"), new element=w258) -> (w257:string[])  [unwired: 1 in]
    }
    frame 1, Default {
      n67 = Insert Into Array(array=w262, new element=string[] ["", "", ""] ("输出数组")) -> (w261:string[])  [unwired: 1 in]
    }
  }
  n68 = Number To Fractional String(number=w13, precision (6)=i16 9 ("精度(6)")) -> (F-format string=w12:string)  [unwired: 2 in]
  n69 = case shown="2" "6221ch" {
    tunnel: w12 -> [w264 w266 w268 w269]
    tunnel: [w264 w265 w267 w270] -> w11
    tunnel: [w263 w266 w267 w270] -> w10
    tunnel: [w263 w265 w268 w270] -> w9
    tunnel: [w263 w265 w267 w269] -> w1
    frame 1, Default {
      w263 = ""
    }
    frame 2 {
      w265 = ""
    }
    frame 3 {
      w267 = ""
    }
    frame 4 {
      w270 = ""
    }
  }
  n70 = case shown="假" w6 {
    tunnel: ["0" "1"] -> w5
    frame False {
    }
    frame True {
    }
  }
  n71 = To Double Precision Float(number=w24) -> (double precision float=w47:dbl)
  n72 = Number To Fractional String(number=w27, precision (6)=i16 6 ("精度(6)")) -> (F-format string=w34:string[])  [unwired: 2 in]
  n73 = Number To Fractional String(number=w47, precision (6)=i16 2 ("精度(6)")) -> (F-format string=w33:string)  [unwired: 2 in]
  n74 = Number To Fractional String(number=w19, precision (6)=i16 0 ("精度(6)")) -> (F-format string=w7:string)  [unwired: 2 in]
  n75 = Number To Fractional String(number="压电陶瓷电压 (Vpp)", precision (6)=i16 0) -> (F-format string=w32:string)  [unwired: 2 in]
  n76 = Number To Fractional String(number=w14, precision (6)=i16 12) -> (F-format string=w8:string)  [unwired: 2 in]
  n77 = Build Array (concatenate)(w33, w34, w32, w2, w2, w15, w11, w10, w9, w1, w8, w7, w5) -> (→"数组":string[])
  "错误输出" <- w23
  "输出簇" <- w22
